vi "Simplify_ONE_Mult_Assign.vi"(8 "Assignment Statement":i32, 11 "Parse Tree in":T1[](array[typedef])) -> (3 "Parse Tree":T1[](array[typedef]))   [LabVIEW 2021]
uses:
  <resource>/MathScriptParser/Statement.ctl
  <resource>/MathScriptParser/NodeType.ctl
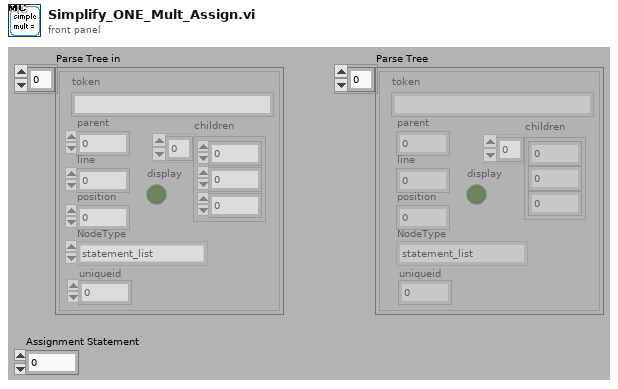
[diagram p1: front panel]
types:
  T1 = typedef "Statement.ctl" = cluster{"parent":u32, "children":u32[], "token":string, "NodeType":T2, "line":u32, "display":bool, "position":u32, "uniqueid":u32}
  T2 = typedef "NodeType.ctl" = enum16{"statement_list", "expression_list", "matrix", "row", "command", "function_1_1", "function_1_N", "function_N_1", "function_N_N", "operator", "assignment", "for", "if", "switch", "while", "try", "range", "identifier", "struct_field", "constant", "udfunction_1_1", "udfunction_1_N", "udfunction_N_1", "udfunction_N_N", "udfunction_0_0", "udfunction_0_1", "udfunction_0_N", "udfunction_1_0", "udfunction_N_0", "function_0_1", "function_0_N", "struct_ref", "array_ref", "cell_array_ref", "cell_matrix"}
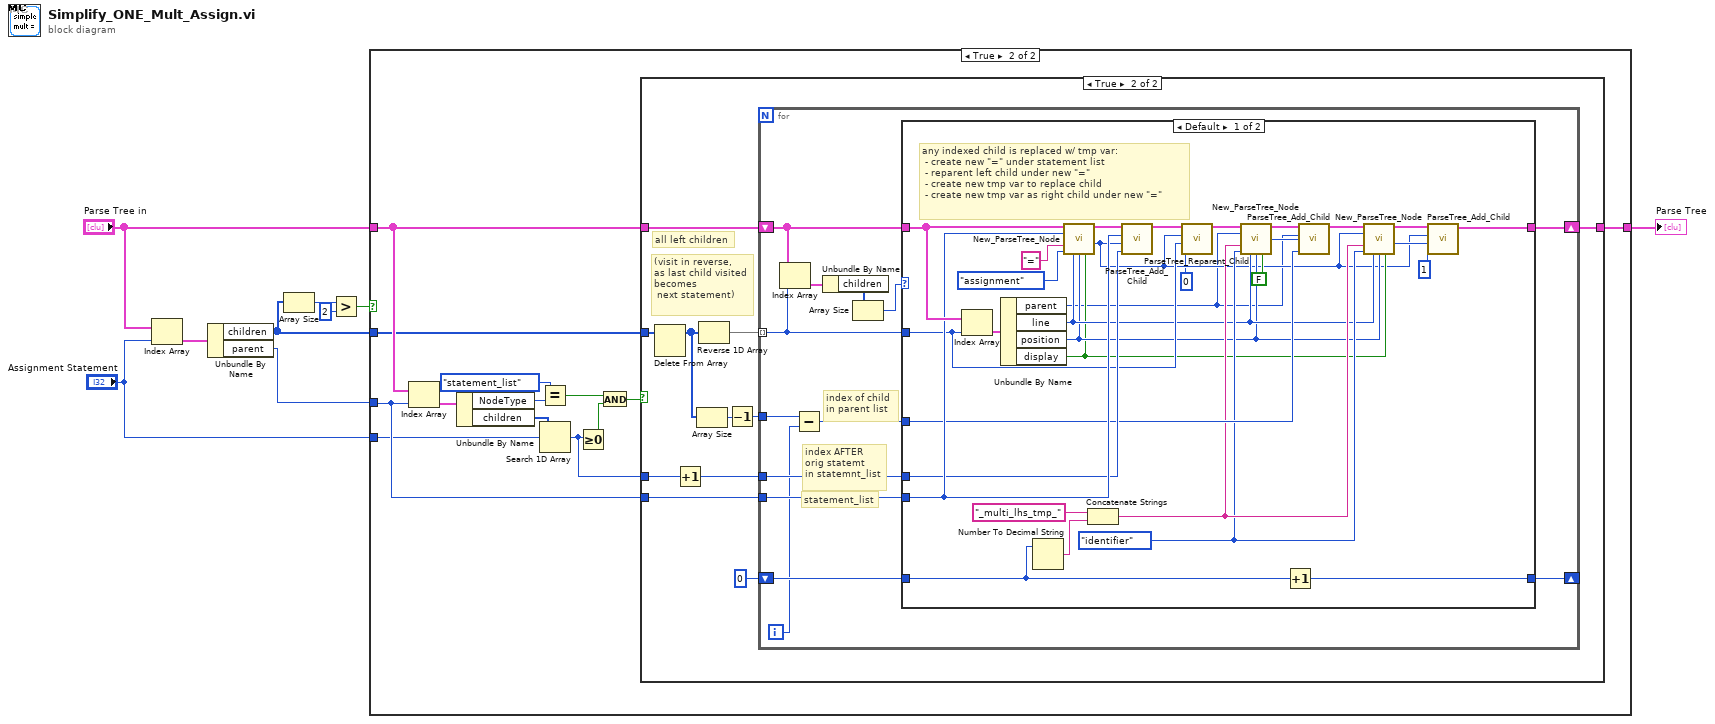
[diagram p0: block diagram]
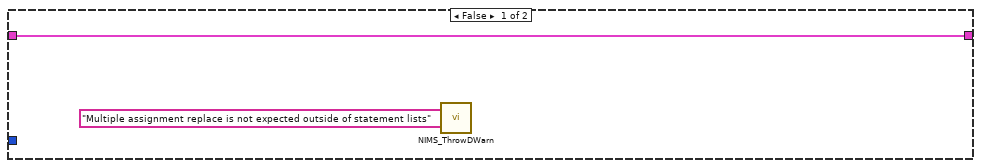
[diagram p3: hidden frame]
diagram:
  n1 = Index Array(array="Parse Tree in", index="Assignment Statement") -> (element=w9:T1)
  n2 = Unbundle By Name(w9) -> ("children"=w5:u32[], "parent"=w6:u32)
  n3 = Array Size(array=w5) -> (size(s)=w8:i32)
  n4 = Greater?(x=w8, y=2) -> (0:w4:bool)
  n5 = case shown="True" w4 {
    tunnel: w5 -> [_ w13]
    tunnel: w6 -> [_ w12]
    tunnel: "Parse Tree in" -> [w10 w15]
    tunnel: [w10 w14] -> w2
    tunnel: "Assignment Statement" -> [_ w11]
    frame False {
    }
    frame True {
      n6 = Index Array(array=w15, index=w12) -> (element=w18:T1)
      n7 = Unbundle By Name(w18) -> ("NodeType"=w19:T2, "children"=w21:u32[])
      n8 = Equal?(x=NodeType."statement_list", y=w19) -> (x = y?=w23:bool)
      n9 = Search 1D Array(1D array=w21, element=w11) -> (index of element=w16:i32)  [unwired: 1 out]
      n10 = Greater Or Equal To 0?(x=w16) -> (x >= 0?=w22:bool)
      n11 = And(x=w23, y=w22) -> (x .and. y?=w17:bool)
      n12 = case shown="True" w17 {
        tunnel: w13 -> [_ w36]
        tunnel: w16 -> [_ w33]
        tunnel: w12 -> [_ w32]
        tunnel: w15 -> [w25 w35]
        tunnel: [w25 w34] -> w14
        frame False {
          n13 = call <vilib>:"NIMS_ThrowDWarn.vi"("DWarn"="Multiple assignment replace is not expected outside of statement lists") -> ()  [unwired: 1 in]
        }
        frame True {
          # "(visit in reverse,\nas last child visited\nbecomes\n next statement)"
          # "all left children"
          n14 = Delete From Array(array=w36) -> (array with subset deleted=w28:u32[])  [unwired: 2 in, 1 out]
          n15 = Increment(x=w33) -> (x+1=w30:i32)
          n16 = Array Size(array=w28) -> (size(s)=w27:i32)
          n17 = Reverse 1D Array(array=w28) -> (reversed array=w29:u32[])
          n18 = Decrement(x=w27) -> (x-1=w26:i32)
          n19 = for {
            tunnel: w29 -> [w46] mode=indexing
            shift-right: [w47] -> w34
            shift-left: w35 -> [w48]
            tunnel: w30 -> [w45]
            tunnel: w32 -> [w44]
            shift-right: [w42] -> _
            shift-left: 0 -> [w43]
            tunnel: w26 -> [w41]
            i -> [w40]
            # "index of child\nin parent list"
            # "statement_list"
            # "index AFTER \norig statemt\nin statemnt_list"
            n20 = Index Array(array=w48, index=w46) -> (element=w49:T1)
            n21 = Subtract(x=w41, y=w40) -> (x-y=w39:i32)
            n22 = Unbundle By Name(w49) -> ("children"=w38:u32[])
            n23 = Array Size(array=w38) -> (size(s)=w37:i32)
            n24 = case shown="Default" w37 {
              tunnel: [w53 w82] -> w47
              tunnel: w48 -> [w79 w82]
              tunnel: w46 -> [w74 _]
              tunnel: w45 -> [w76 _]
              tunnel: w44 -> [w77 _]
              tunnel: w43 -> [w67 w81]
              tunnel: [w66 w81] -> w42
              tunnel: w39 -> [w65 _]
              frame Default {
                w62 = NodeType."identifier" ("NodeType")
                # "any indexed child is replaced w/ tmp var:\n - create new \"=\" under statement list\n - reparent left child under new \"=\"\n - create new tmp var to replace child \n - create new tmp var as right child under new \"=\""
                n25 = Index Array(array=w79, index=w74) -> (element=w80:T1)
                n26 = Unbundle By Name(w80) -> ("parent"=w52:u32, "line"=w61:u32, "position"=w60:u32, "display"=w59:bool)
                n27 = Number To Decimal String(number=w67) -> (decimal integer string=w69:string)  [unwired: 1 out]
                n28 = call <vilib>:"New_ParseTree_Node.vi"("Parse Tree in"=w79, "parent"=w77, "token"="=", "NodeType"=NodeType."assignment", "line"=w61, "position"=w60, "display"=w59) -> ("Parse Tree out"=w78:T1[], "new node index"=w55:i32)  [unwired: 6 in, 1 out]
                n29 = Concatenate Strings("_multi_lhs_tmp_" ("string"), w69) -> (w63:string)
                n30 = call <vilib>:"ParseTree_Add_Child.vi"("index of child"=w76, "child"=w55, "parent"=w77, "Parse Tree in"=w78) -> ("Parse Tree out"=w75:T1[])  [unwired: 7 out]
                n31 = call <vilib>:"ParseTree_Reparent_Child.vi"("index of child in new parent"=0, "child"=w74, "new parent"=w55, "Parse Tree in"=w75) -> ("Parse Tree out"=w72:T1[])  [unwired: 7 out]
                n32 = call <vilib>:"New_ParseTree_Node.vi"("Parse Tree in"=w72, "parent"=w52, "token"=w63, "NodeType"=w62, "line"=w61, "position"=w60, "display"=FALSE) -> ("Parse Tree out"=w73:T1[], "new node index"=w68:i32)  [unwired: 6 in, 1 out]
                n33 = Increment(x=w67) -> (x+1=w66:i32)
                n34 = call <vilib>:"ParseTree_Add_Child.vi"("index of child"=w65, "child"=w68, "parent"=w52, "Parse Tree in"=w73) -> ("Parse Tree out"=w64:T1[])  [unwired: 7 out]
                n35 = call <vilib>:"New_ParseTree_Node.vi"("Parse Tree in"=w64, "parent"=w55, "token"=w63, "NodeType"=w62, "line"=w61, "position"=w60, "display"=w59) -> ("Parse Tree out"=w56:T1[], "new node index"=w57:i32)  [unwired: 6 in, 1 out]
                n36 = call <vilib>:"ParseTree_Add_Child.vi"("index of child"=1, "child"=w57, "parent"=w55, "Parse Tree in"=w56) -> ("Parse Tree out"=w53:T1[])  [unwired: 7 out]
              }
              frame 0 {
                # "simple writes to identifiers remain unchanged"
              }
            }
          }
        }
      }
    }
  }
  "Parse Tree" <- w2
